vi "Main Tclk.vi"() -> ()   [LabVIEW 2018] (continued)
  in  "Hardware Configuration":T25={"SEM X coil"="SEM-X", "SEM Y coil"="SEM-Y", "FIB X coil"="FIB/ao0", "FIB Y coil"="FIB/ao1", "FIB Detector"="FIB/ai1", "SEM Detectors"="Detectors", "Det min (V)"=-10.0, "Det max (V)"=10.0, "Eanable COM"=TRUE, "COM port"="COM1", "FIB Beam blank"="FIB/port0/line0", "FIB Ext Scan"="FIB/port0/line1", "Det. FIB-NI auto switch"="FIB/port0/line2", "Shutter Drive"="Log/ao0", "Machine Type"=2, "FIB Faraday Cup"="FIB/ai3", "Configuration file"=path "D:/3D FIB-SEM Files/Jeiss.ini", "SEM Max FOV (um)"=350.0, "Machine ID"="Jeiss6/Merlin-xxxx", "Save config file"=FALSE, "Temperature port"="COM3", "Brightness A"=35.0, "Contrast A"=28.0, "Detector B name"="ESB @ 600 V", "Brightness B"=30.0, "Contrast B"=38.0, "Logging Device"="Log"} {"Machine Type" items=["Feiss", "NVision", "Jeiss"]}
  in  "Api":refnum<k7>(container)
  in  "SEM Scan Parameters":T26={"X size (um)"=80.0, "Y size (um)"=80.0, "X center (um)"=0.0, "Y center (um)"=0.0, "X size (V)"=3.2324881417410714, "X size auto"=TRUE, "X stig"=[[0.0]], "Y stig"=[[0.0]], "X aln"=[[0.0]], "Y aln"=[[0.0]], "Scan rate (Hz)"=10000000, "Oversampling"=2, "Oversampling auto"=TRUE, "Frame line rampdown ratio"=0.1, "Pixel size (nm)"=8.0, "WD (mm)"=[[3.0]], "X tiles"=1, "Y tiles"=1, "Overlap (um)"=2.0, "Interlaced"=FALSE, "dX (um)"=[0.0], "dY (um)"=[0.0], "Frames"=1} {"dY (um)" format="%.1f"; "dX (um)" format="%.1f"; "Frames" min=1 step=1; "WD (mm)" step=0.001 format="%.4f"; "Y aln" format="%.1f"; "X aln" format="%.1f"; "Y stig" format="%.1f"; "X stig" format="%.1f"; "Overlap (um)" min=0 step=1; "Y tiles" min=1; "X tiles" min=1; "X size (um)" min=0 format="%.2f"; "Y size (um)" min=0 format="%.2f"; "Frame line rampdown ratio" min=0 max=1 step=0.05 format="%.2g"; "X center (um)" step=1 format="%.3f"; "Y center (um)" step=1 format="%.3f"; "X size (V)" format="%_4g"; "Scan rate (Hz)" max=4000000 step=100000 format="%.2e"; "Pixel size (nm)" min=0.1}
  in  "SEM Options":T27={"GetInfo"=TRUE, "Set Det A para"=TRUE, "Set WD"=FALSE, "Set Mag"=TRUE, "Set stig"=FALSE, "Set aln"=FALSE, "Display"=TRUE, "Save"=TRUE, "8-bit"=FALSE, "Detector A"=TRUE, "Detector B"=TRUE, "Detector C"=FALSE, "Detector D"=FALSE, "Inverse A"=FALSE, "Inverse B"=FALSE, "Inverse C"=FALSE, "Inverse D"=FALSE, "Inverse PNG"=TRUE, "Freeze"=TRUE, "PNG only"=FALSE, "Upload"=FALSE, "Delete after upload"=FALSE}
  in  "Focus Index Options":T28={"Keep aspect ratio"=FALSE, "Show Focus Index"=TRUE, "Focus Index primary grid center"=TRUE, "X Grids"=[[1]], "Y Grids"=[[1]], "Primary X index"=[[1]], "Primary Y index"=[[1]]} {"Y Grids" step=2; "X Grids" step=2}
  out "AS Count":u8 caption="Counts"
  out "AF Count":u8 caption="Counts"
  in  "AS Steps":u8=7
  in  "AS Range (%)":sgl=0.4 min=0 step=1
  in  "Auto Stig":bool
  in  "FI Detector":u16(ring) caption="Detector" items=["A", "B", "C", "D"]
  in  "Auto Focus":bool
  in  "AF Range (nm)":sgl=1800.0 caption="Range" min=0 step=1000
  in  "AF Steps":u8=7 caption="Steps"
  in  "Auto Optimzation":bool=TRUE
  in  "Images per Auto Optimization":u16=200 caption="Auto Optimization Every"
  in  "AA Steps":u8=7
  in  "AA Range (%)":sgl=18.0
  in  "Auto Align":bool
  out "AA Count":u8 caption="Counts"
  in  "Y shift (nm/image)":sgl step=0.1 format="%.1f"
  in  "X shift (nm/image)":sgl step=0.1 format="%.1f"
  in  "Mid Mag SEM":T29={"Mid mag scan"=FALSE, "Prior to main scan"=FALSE, "Mid mag interval"=500, "X size (um)"=200.0, "Y size (um)"=200.0, "X center (um)"=0.0, "Y center (um)"=0.0, "Mid mag scan rate (Hz)"=1000000, "Pixel size (nm)"=10.0, "Show MM box"=TRUE} {"X center (um)" step=1.0 format="%.4f"; "Y center (um)" step=1.0 format="%.4f"; "Mid mag interval" min=1 step=1; "Mid mag scan rate (Hz)" max=4000000 step=100000 format="%.2e"}
  in  "Low Mag SEM":T30={"Low mag scan"=TRUE, "Prior to main scan"=FALSE, "Low mag interval"=1, "Low mag scan FOV (micron)"=300.0, "Low mag scan rate (Hz)"=1000000, "Show HM box"=TRUE} {"Low mag interval" min=1 step=1; "Low mag scan rate (Hz)" max=4000000 step=100000 format="%.2e"; "Low mag scan FOV (micron)" step=50.0}
  out "Mid Mag SEM on":bool
  in  "Manual Upload":bool
  in  "Smart upload":bool=TRUE
  in  "Smart upload FI threshold":u8=75 caption="Threshold"
  in  "Start Current DataLog":bool
  in  "Interval (s)":u16=60
  in  "Start FIB HV DataLog":bool=TRUE
  out "Logging Channels":tag[](array[tag])=["Log/ai0", "Log/ai1", "Log/ai2", "Log/ai3", "Log/ai4", "Log/ai5", "Log/ai6", "Log/ai7", "Log/ai8", "Log/ai9", "Log/ai10", "Log/ai11", "Log/ai12", "Log/ai13", "Log/ai14", "Log/ai15", "Log/ai16", "Log/ai17", "Log/ai18", "Log/ai19", "Log/ai20", "Log/ai21", "Log/ai22", "Log/ai23", "Log/ai24", "Log/ai25", "Log/ai26", "Log/ai27", "Log/ai28", "Log/ai29", "Log/ai30", "Log/ai31"]
  in  "Parameter Names":string[](array[string])=["Faraday Cup Current", "Specimen Current", "Beam Dump 1 Current", "Beam Dump 2 Current"]
  in  "Samples size":u16=100
  out "Log Device":tag="Log"
  in  "Sample rate (Hz)":dbl=1000.0 format="%0.2f"
  in  "Enable logging":bool=TRUE
  out "Active logging channels":string="Log/ai0:3"
  out "Re-read HVDataLog":bool caption="Success"
  out "Logging status before profiling":bool
  in  "File Information":T31={"File path"=path "E:/Images", "Notes"="", "Save recipe"=FALSE, "Load recipe"=FALSE, "Sample ID"=""}
  in  "After SEM":bool=TRUE
  in  "Save Probe Table":bool
  in  "Max FIB probe":bool
  in  "Min FIB probe":bool
  in  "SEM Shutter":bool
  in  "Extractor (kV)":sgl=-6.3 step=0.01 format="%.3f"
  in  "Sweep enabled":bool
  in  "Focus (V)":dbl min=-10.0 max=10.0 step=0.1 format="%.3g"
  in  "Sweep rate (Hz)":dbl=0.5 min=0.01 step=0.1 format="%0.2f"
  in  "Imbalance (V)":dbl min=-10.0 max=10.0 step=0.1 format="%.3g"
  in  "Sweep direction":bool
  in  "Angle (V)":dbl min=-10.0 max=10.0 step=0.1 format="%.3g"
  in  "Position (V)":dbl min=-10.0 max=10.0 step=0.1 format="%.3g"
  in  "Level #":u8
  in  "Sweep #":u8=1 min=1
  in  "FIB Scan Parameters":T32={"X resolution"=512, "Z resolution"=512, "X center"=0.0, "Z center"=0.0, "X size (V)"=16.0, "Z size (V)"=16.0, "Frame line rampdown ratio"=-0.1, "Scan rate (Hz)"=2000000, "Oversampling"=2} {"Z size (V)" min=0.0 max=20.0; "X size (V)" min=0.0 max=20.0; "Frame line rampdown ratio" min=-1.0 max=1.0 step=0.05 format="%.2g"; "Scan rate (Hz)" max=4000000 format="%#.6p"; "Z resolution" max=2048; "X resolution" max=2048}
  in  "FIB Options":T33={"Scan mode"=0, "Flip x"=FALSE, "Flip z"=TRUE, "Det"=0} {"Scan mode" items=["Raster", "Serpentine"]; "Det" items=["Detector A", "Detector B"]}
  in  "Update":bool
  in  "FIB-SEM Angle":dbl=90.0 min=0.0 max=90.0
  in  "FIB Zoom Parameters":T34={"X resolution"=500, "Y resolution"=50, "X center"=0.0, "Y center"=0.0, "X size (V)"=0.0, "Y size (V)"=0.0, "Frame line rampdown ratio"=-0.1, "Scan rate (Hz)"=2000000, "Oversampling"=2} {"Frame line rampdown ratio" min=-1.0 max=1.0 step=0.05 format="%.2g"; "Scan rate (Hz)" max=4000000 format="%#.6p"}
  in  "FIB Bit Size (nm)":dbl
  in  "FIB time lapse (s)":u32=60
  out "FIB file name":path
  in  "SEM-FIB Delay (s)":u32
  in  "FIB Y zoom pixel (nm)":dbl=20.0 caption="Y pixel (nm)" format="%.1f"
  in  "Pre image":bool
  in  "Post image":bool
  out "13nA Condenser (V)":i32=565
  out "27nA Condenser (V)":i32=585
  out "FIB probe switching":string="Go to                 or               current of the same probe "
  out "Fail #":u8
  out "SEM shutter status":string="Unknown"
  in  "FIB Imaging Probe":string(combo)="30kV:50pA ref"
  in  "Damping":bool
  in  "Shtr Tune":bool
  in  "Stop Reheat":bool
  in  "Reheat Parameters":T1={"Filament I (A)"=3.0, "Reheat time (s)"=45.0, "Emission (uA)"=1.5, "Calculate V/I slope"=TRUE, "Pre-calc delay (min)"=5.0, "Disable Reheat Retries"=FALSE, "Restore Voltages"=TRUE} {"Pre-calc delay (min)" format="%.2f"; "Emission (uA)" format="%.1f"; "Filament I (A)" format="%.2f"; "Reheat time (s)" format="%.1f"}
  out "Auto reheat running":bool
  out "Last auto reheat":timestamp
  out "Reheat complete file":path=path "C:/Program Files (x86)/FEI Company/BDS/Reheat/Complete.txt"
  out "Reheat stopped file":path=path "C:/Program Files (x86)/FEI Company/BDS/Reheat/Stopped.txt"
  out "FIB Reheat Log Files":path=path "D:/3D FIB-SEM Files/FIB Reheat Log"
  out "Reheat time":timestamp
  out "Reheat start file":path=path "C:/Program Files (x86)/FEI Company/BDS/Reheat/Start.txt"
  out "Shutter Drive Local?":tag="Log/ao0"
  out "Send reheat start email":bool
  in  "Open FIB gun valve":bool=TRUE caption="Gun Valve"
  out "FIB Gun Valve Status":string="FIB Gun Valve is Open"
  out "FIB Gun State":string="Regulating"
  in  "Request to stop reheat":bool
  in  "Request to reheat":bool
  out "Reheat completed":bool
  in  "Turn FIB gun standby":bool
  in  "Turn off FIB gun":bool
  in  "Turn on FIB gun":bool=TRUE
  out "FIB V/I slope":sgl format="%.1f"
  in  "Get V/I slope":bool
  in  "FIB probe auto min":bool
  in  "FIB Milling Objective (V)":sgl=14275.0
  in  "FIB Profile":bool
  in  "Reset Focus":bool=TRUE
  in  "Mill Stop":bool
  in  "Mill Manual Pause":bool
  in  "Beam blanked":bool
  in  "Spot":bool
  in  "Milling para":T35={"X resolution"=4096, "Z resolution"=125001, "X offset (um)"=0.0, "Z offset (um)"=0.0, "X center (um)"=0.0, "Z center (um)"=0.0, "X size (um)"=250.0, "Z size (um)"=250.0, "UL-Ang"=90.0, "UR-Ang"=90.0, "Line milling time (s)"=5.0, "Z-step (nm)"=8.0, "Lines auto pause"=1, "Auto pause"=FALSE, "Mill from Bottom"=FALSE, "FIB FOV (um)"=500.0, "Auto Profile"=FALSE, "Mill start from Last"=FALSE, "FIB PID on"=FALSE, "FIB PID reset"=FALSE, "FIB PID measured"=0, "FIB PID target"=0.0, "FIB PID target slope"=0.0, "FIB PID P"=0.001, "FIB PID I"=0.01, "FIB PID D"=0.0, "Emission (uA)"=1.36, "Suppressor (V)"=50.0, "Auto reheat"=FALSE} caption="Milling Parameters" {"Suppressor (V)" step=0.1; "Emission (uA)" step=0.1 format="%.2g"; "FIB PID measured" items=["Spec.", "B.D. 1", "B.D. 2", "Mill", "Spec. +"]; "FIB PID target slope" min=-1 max=1 step=0.1; "FIB PID target" step=0.1 format="%.1f"; "UR-Ang" format="%.2f"; "UL-Ang" format="%.2f"; "Z offset (um)" step=0.02 format="%.3g"; "X offset (um)" step=1 format="%.3g"; "FIB FOV (um)" format="%.3g"; "Line milling time (s)" step=0.1 format="%.1f"; "Z center (um)" format="%#.3g"; "X center (um)" format="%#.3g"}
  in  "Mill":bool
  in  "ROI":bool
  in  "Stig Options":enum16{"Defaut", "Stig X", "Stig Y"}(ring)
  in  "Transition time (min)":u16
  in  "PID Target (%)":sgl=100.0 format="%.1f"
  in  "FIB Milling Probe":string(combo)="30kV:50pA ref"
  in  "FIB blank condenser %":u8=50 caption="FIB Condenser @ SEM:" max=100
  in  "Additional Info":cluster{"Restart flag":u8, "Stage move flag":u8}
  in  "Coarse milling":bool
  out "Temperature warning armed":bool
  in  "E-mail test":bool
  out "3D image paused armed":bool=TRUE
  in  "Mail server":string="mail.hhmi.org"
  in  "Email Alert Recipients":string[](array[string])=["xuc@janelia.hhmi.org"]
  out "FIB emission limit warning armed":bool=TRUE
  out "EHT off":bool
  out "SW error warning armed":bool=TRUE
  out "Focus index warning armed":bool=TRUE
  out "Focus index recovery active":bool
  out "Temperature recovery active":bool
  in  "Alert Settings":T36={"3D imaging paused alarm"=TRUE, "FIB emission warning"=TRUE, "Low limit"=1.38, "High limit"=2.0, "Specimen @ SEM alarm"=TRUE, "FIB CL current alarm"=TRUE, "Beam Dump 1 alarm"=TRUE, "Milling Z voltage alarm"=TRUE, "EHT off alarm"=TRUE, "Detector over scale warning"=TRUE, "Image clipping alarm"=FALSE, "Warning limit (um)"=1.5, "Stop limit (um)"=0.5, "Temperature alarm"=TRUE, "Pause 3D-ING"=FALSE, "Low limit (F)"=65.0, "High limit (F)"=80.0, "Temp limit auto"=TRUE, "Delta (F)"=0.2, "Gradient limit (F/min)"=0.03, "SW error warning"=TRUE, "Focus index warning"=TRUE, "Focus index low limit"=0.1, "Focus index stop limit"=0.0, "Run Auto Stig"=FALSE, "FI low limit auto"=TRUE, "FI stop limit auto"=TRUE} {"Stop limit (um)" format="%.2f"; "Warning limit (um)" format="%.2f"; "Focus index stop limit" format="%_3g"; "Focus index low limit" format="%_3g"; "High limit (F)" format="%.2g"; "Low limit (F)" format="%.2g"; "High limit" format="%.2f"; "Low limit" format="%.2f"}
  out "Reheat warning armed":bool=TRUE
  out "Email Log Files":path=path "D:/3D FIB-SEM Files/Email Log"
  out "Initial Options":T27={"GetInfo"=TRUE, "Set Det A para"=TRUE, "Set WD"=FALSE, "Set Mag"=TRUE, "Set stig"=FALSE, "Set aln"=FALSE, "Display"=TRUE, "Save"=TRUE, "8-bit"=TRUE, "Detector A"=TRUE, "Detector B"=TRUE, "Detector C"=FALSE, "Detector D"=FALSE, "Inverse A"=FALSE, "Inverse B"=FALSE, "Inverse C"=FALSE, "Inverse D"=FALSE, "Inverse PNG"=TRUE, "Freeze"=TRUE, "PNG only"=TRUE, "Upload"=TRUE, "Delete after upload"=FALSE}
  in  "Scan xn":bool
  out "Status message":string="API Initialized"
  in  "FIB":bool
  out "COM port":refnum<visa-resource-name>="COM1"
  in  "Image Tabs":T37(tab)=enum."Auto Focus / Stig / Align"
  out "Det B LM":i16[][](graph)
  out "Det A LM":i16[][](graph)
  out "Det B":i16[][](graph)
  out "Det A":i16[][](graph)
  out "Low res scale tiled":dbl[][](array[numeric])
  in  "Tiled Image fit to":u8(ring) items=["Width", "Height"]
  out "Det A over scale":bool caption="Over scale"
  out "Det B over scale":bool caption="Over scale"
  out "DetA e- Scaling":sgl caption="Electon # Scaling" format="%.3g"
  out "Detector A":i16[][](graph) caption="InLens"
  out "Detector B":i16[][](graph) caption="ESB @ 600 V"
  out "DetB e- Scaling":sgl caption="Electon # Scaling" format="%.3g"
  out "Detector A Low Mag":i16[][](graph)
  out "Detector B Low Mag":i16[][](graph)
  out "FIB Image":i16[][](graph)
  out "Faraday Cup RT":sgl caption="Faraday Cup" format="%.3g"
  out "Specimen RT":sgl=5.58914 caption="Specimen" format="%.3g"
  out "BD1 RT":sgl=5.6069436 caption="Beam Dump" format="%.3g"
  out "BD2 RT":sgl=5.6180186 format="%.3g"
  out "Cursor Z (V)":dbl format="%.4g"
  out "Post Image":i16[][](graph)
  out "Pre Image":i16[][](graph)
  out "FIB Y zoom size (um)":dbl caption="Y size (um)" format="%.3g"
  out "FIB X zoom size (um)":dbl caption="Y size (um)" format="%.3g"
  out "AAX Success tiled":bool[][](array[boolean]) caption="Success"
  out "AAY Y tile":u8 caption="Y" min=1
  out "AAY X tile":u8 caption="X" min=1
  out "ASY Y tile":u8 caption="Y" min=1
  out "ASY X tile":u8 caption="X" min=1
  out "AAX Y tile":u8 caption="Y" min=1
  out "AAX X tile":u8 caption="X" min=1
  out "ASX Y tile":u8 caption="Y" min=1
  out "ASX X tile":u8 caption="X" min=1
  out "AF Y tile":u8 caption="Y" min=1
  out "AF X tile":u8 caption="X" min=1
  out "Auto Aln Y":T38(graph)
  out "Auto Aln X":T38(graph)
  out "Dynamic Focus":cluster{cluster{sgl, "Numeric":dbl}[]}[](graph)
  out "Auto Stig Y":T38(graph)
  out "Auto Stig X":T38(graph)
  out "FI array":sgl[](array[numeric])
  out "Auto Focus Graph":T38(graph)
  out "FI grid array":sgl[][][](array[numeric])
  out "WD array tiled":sgl[][][](array[numeric])
  out "AF Success tiled":bool[][](array[boolean]) caption="Success"
  out "ASX Success tiled":bool[][](array[boolean]) caption="Success"
  out "ASY Success tiled":bool[][](array[boolean]) caption="Success"
  out "AAY Success tiled":bool[][](array[boolean]) caption="Success"
  out "Best WD (mm) tiled":dbl[][](array[numeric]) caption="Best WD (mm)" format="%.4g"
  out "Best WD FI tiled":dbl[][](array[numeric]) format="%#_3g"
  out "Best Stig X (%) tiled":dbl[][](array[numeric]) caption="Best Stig X (%)" format="%.2g"
  out "Best Stig X FI tiled":dbl[][](array[numeric]) format="%#_3g"
  out "Best Stig Y (%) tiled":dbl[][](array[numeric]) caption="Best Stig Y (%)" format="%.2g"
  out "Best Stig Y FI tiled":dbl[][](array[numeric]) format="%#_3g"
  out "Best Aln X (%) tiled":dbl[][](array[numeric]) caption="Best Aln X (%)" format="%.2g"
  out "Best Aln X FI tiled":dbl[][](array[numeric]) format="%#_3g"
  out "Best Aln Y (%) tiled":dbl[][](array[numeric]) caption="Best Aln Y (%)" format="%.2g"
  out "Best Aln Y FI tiled":dbl[][](array[numeric]) format="%#_3g"
  out "Slope tiled":dbl[][](array[numeric]) caption="Slope" format="%#_4g"
  out "Focus index log":cluster{u32[], "Focus index array":sgl[]}[](graph)
  out "Delta X log":T39(graph)
  out "Delta Z log":T40(graph)
  out "Delta Y log":T41(graph)
  out "Beam Dump log":cluster{u32[], "BD1 low limit array":sgl[]}[](graph)
  out "Specimen I log":cluster{u32[], "SEM Specimen I array":sgl[]}[](graph)
  out "Faraday Cup log":cluster{u32[], "Temp low limit array":sgl[]}[](graph)
  out "Temp log":cluster{u32[], "Temp array":sgl[]}[](graph)
  out "Log time array":u32[](array[numeric])
  out "FIB HV DataLog":cluster{sgl, sgl}(graph)={849.284, 1.5152843}
  out "Measurements":sgl[][](graph)=[[0.0, 0.0, 0.0, 0.0, 0.0, 0.0, 0.0, 0.0, 0.0, 0.0, 0.0, 0.0, 0.0, 0.0, 0.0, 0.0, 0.0, 0.0, 0.0, 0.0, 0.0, 0.0, 0.0, 0.0, 0.0, 0.0, 0.0, 0.0, 0.0, 0.0, 0.0, 0.0, 0.0, 0.0, 0.0, 0.0, 0.0, 0.0, 0.0, 0.0, 0.0, 0.0, 0.0, 0.0, 0.0, 0.0, 0.0, 0.0, 0.0, 0.0, 0.0, 0.0, 0.0, 0.0, 0.0, 0.0, 0.0, 0.0, 0.0, 0.0, 0.0, 0.0, 0.0, 0.0, 0.0, 0.0, 0.0, 0.0, 0.0, 0.0, 0.0, 0.0, 0.0, 0.0, 0.0, 0.0, 0.0, 0.0, 0.0, 0.0, 0.0, 0.0, 0.0, 0.0, 0.0, 0.0, 0.0, 0.0, 0.0, 0.0, 0.0, 0.0, 0.0, 0.0, 0.0, 0.0, 0.0, 0.0, 0.0, 0.0], [5.6226387, 5.0222063, 5.522835, 5.619419, 5.61137, 5.606541, 5.603322, 5.603322, 5.603322, 5.600102, 5.603322, 5.604931, 5.6017118, 5.600102, 5.600102, 5.596883, 5.6017118, 5.5984926, 5.5984926, 5.5984926, 5.5984926, 5.600102, 5.5984926, 5.5984926, 5.600102, 5.5984926, 5.5984926, 5.600102, 5.595273, 5.596883, 5.5984926, 5.595273, 5.600102, 5.595273, 5.595273, 5.595273, 5.595273, 5.593663, 5.593663, 5.595273, 5.593663, 5.5920534, 5.595273, 5.5920534, 5.595273, 5.596883, 5.595273, 5.595273, 5.595273, 5.593663, 5.595273, 5.596883, 5.595273, 5.593663, 5.593663, 5.593663, 5.596883, 5.593663, 5.5920534, 5.593663, 5.5920534, 5.593663, 5.5920534, 5.5920534, 5.593663, 5.5904436, 5.5920534, 5.593663, 5.5904436, 5.593663, 5.595273, 5.5920534, 5.5920534, 5.593663, 5.5904436, 5.5920534, 5.5904436, 5.5920534, 5.5904436, 5.5904436, 5.5920534, 5.5920534, 5.5920534, 5.5904436, 5.5920534, 5.5920534, 5.5872245, 5.595273, 5.5904436, 5.5904436, 5.5904436, 5.5920534, 5.588834, 5.5904436, 5.5904436, 5.5920534, 5.5920534, 5.5904436, 5.588834, 5.5904436], [6.6013584, 5.604931, 5.519615, 5.5920534, 5.608151, 5.608151, 5.606541, 5.608151, 5.604931, 5.604931, 5.606541, 5.603322, 5.6017118, 5.603322, 5.6017118, 5.603322, 5.604931, 5.603322, 5.603322, 5.603322, 5.6017118, 5.6017118, 5.603322, 5.600102, 5.600102, 5.603322, 5.5984926, 5.596883, 5.6017118, 5.596883, 5.5984926, 5.600102, 5.600102, 5.6017118, 5.600102, 5.5984926, 5.6017118, 5.5984926, 5.596883, 5.5984926, 5.596883, 5.5984926, 5.596883, 5.600102, 5.596883, 5.595273, 5.595273, 5.5984926, 5.596883, 5.596883, 5.595273, 5.5984926, 5.5984926, 5.5984926, 5.5984926, 5.595273, 5.596883, 5.593663, 5.596883, 5.593663, 5.595273, 5.5984926, 5.595273, 5.595273, 5.593663, 5.593663, 5.596883, 5.595273, 5.593663, 5.595273, 5.596883, 5.593663, 5.593663, 5.5920534, 5.595273, 5.596883, 5.596883, 5.595273, 5.593663, 5.5920534, 5.593663, 5.593663, 5.5904436, 5.595273, 5.593663, 5.593663, 5.5920534, 5.593663, 5.593663, 5.5920534, 5.5920534, 5.593663, 5.5920534, 5.5920534, 5.593663, 5.593663, 5.5920534, 5.595273, 5.593663, 5.595273], [6.177998, 5.91883, 5.6274676, 5.6097603, 5.6178093, 5.619419, 5.6178093, 5.6178093, 5.61459, 5.6161995, 5.61459, 5.61298, 5.6178093, 5.6161995, 5.61459, 5.6161995, 5.61459, 5.6161995, 5.61298, 5.61298, 5.61137, 5.61137, 5.61459, 5.61137, 5.61137, 5.61137, 5.61298, 5.6097603, 5.61298, 5.61298, 5.61459, 5.61298, 5.61137, 5.608151, 5.61459, 5.608151, 5.6097603, 5.6097603, 5.608151, 5.61137, 5.61137, 5.608151, 5.61298, 5.608151, 5.608151, 5.608151, 5.6097603, 5.608151, 5.606541, 5.604931, 5.6097603, 5.61137, 5.6097603, 5.604931, 5.608151, 5.6097603, 5.606541, 5.6097603, 5.608151, 5.606541, 5.604931, 5.6097603, 5.604931, 5.608151, 5.6097603, 5.608151, 5.606541, 5.604931, 5.608151, 5.606541, 5.606541, 5.604931, 5.606541, 5.606541, 5.6097603, 5.604931, 5.606541, 5.604931, 5.604931, 5.603322, 5.604931, 5.603322, 5.606541, 5.603322, 5.603322, 5.603322, 5.603322, 5.603322, 5.604931, 5.606541, 5.604931, 5.603322, 5.603322, 5.606541, 5.604931, 5.603322, 5.603322, 5.606541, 5.6017118, 5.603322]]
  in  "Clear":bool
  in  "Stop":bool
  in  "Scan x1":bool
  # "Direction"
  # "Start\nfrom"
  # "<"
  # "Grids"
  # "Primary"
  # "Recipe"
  # "Det"
  # "after"
  # "Detector A"
  # "Images"
  # "nm"
  # "%"
  # "%"
  # "Direction"
  # "Start\nfrom"
  # "<"
  # "Grids"
  # "Primary"
  # "Det"
  # "after"
  # "Recipe"
  # "Brightness & Contrast (%)"
  # "Detector A"
  # "Brightness & Contrast (%)"
  # "Brightness & Contrast (%)"
  # "Detector A"
  # "Brightness & Contrast (%)"
  # "Currents (nA)"
  # "/"
  # "line(s)"
  # "% of"
  # "%"
  # "Hz"
  # "Scanning time"
  # "m"
  # "s"
  # "Remaining time"
  # "m"
  # "s"
  # "Cycle time (s)"
  # "@"
  # "Scan coils"
  # "Detector"
  # "Brightness & Contrast (%)"
  # "A       InLens"
  # "Images"
  # "nm"
  # "%"
  # "%"
  # "Det"
  # "after"
  # "Grids"
  # "Primary"
  # "% of FI alarm limit"
  # "Recipe"
  # "FIB Zoom Image"
  # "Flip"
  # "recovers in"
  # "min"
  # "% during Milling"
  # "Direction"
  # "Start\nfrom"
  # "@"
  # "<"
  # "or"
  # "<"
  # "Det"
  # "Images fit to"
  # "Images fit to"
  # "Images fit to"
  # "X"
  # "um"
  # ":"
  # "%"
  # ":"
  # ":"
  # ":"
  # ":"
  # "Faraday Cup"
  # "Specimen"
  # "Beam Dump"
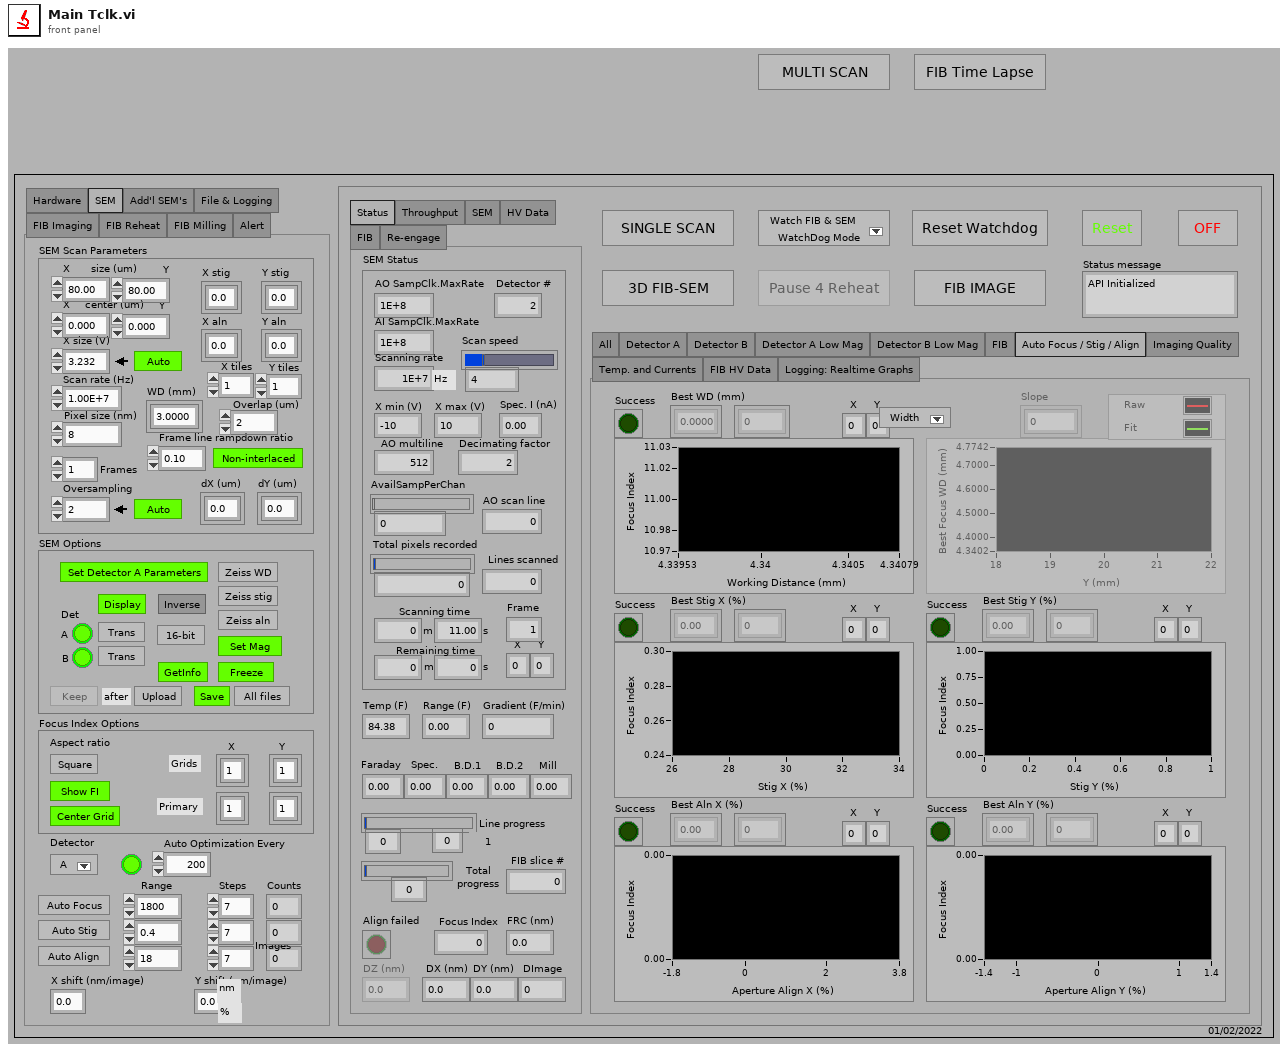
[diagram p1: front panel]
types:
  T1 = cluster{"Filament I (A)":sgl, "Reheat time (s)":sgl, "Emission (uA)":sgl, "Calculate V/I slope":bool, "Pre-calc delay (min)":sgl, "Disable Reheat Retries":bool, "Restore Voltages":bool}
  T2 = cluster{"3D imaging paused alarm":bool, "FIB emission limit warning":bool, "Low limit":dbl, "High limit":dbl, "Specimen @ SEM alarm":bool, "Specimen @ FIB alarm ":bool, "Beam Dump 1 alarm":bool, "Milling Z voltage alarm":bool, "EHT off alarm":bool, "Detector over scale warning":bool, "Image clipping alarm":bool, "Warning limit (um)":sgl, "Stop limit (um)":sgl, "Temperature alarm":bool, "Pause 3D-ING":bool, "Low limit (F)":sgl, "High limit (F)":sgl, "Temp limit auto":bool, "Delta (F)":sgl, "Gradient limit (F/min)":sgl, "SW error warning":bool, "Focus index warning":bool, "Focus index low limit":sgl, "Focus index stop limit":sgl, "Run Auto Stig":bool, "FI low limit auto":bool, "FI stop limit auto":bool}
  T3 = cluster{"dWD":sgl[][], "dX stig":sgl[][], "dY stig":sgl[][], "dX aln":sgl[][], "dY aln":sgl[][], "dX (um)":sgl[], "dY (um)":sgl[]}
  T4 = cluster{cluster{"Center":dbl, "A Img Focus Index":dbl}[]}[][][]
  T5 = cluster{"X size (um)":sgl, "Y size (um)":sgl, "X center (um)":dbl, "Y center (um)":dbl, "X size (V)":dbl, "X size auto":bool, "X stig":sgl[][], "Y stig":sgl[][], "X aln":sgl[][], "Y aln":sgl[][], "Scan rate (Hz)":u32, "Oversampling":u32, "Oversampling auto":bool, "Frame line rampdown ratio":sgl, "Pixel size (nm)":sgl, "WD (mm)":sgl[][], "X tiles":u8, "Y tiles":u8, "Overlap (um)":sgl, "Interlaced":bool, "dX (um)":sgl[], "dY (um)":sgl[], "Frames":u8}
  T6 = cluster{"HW Config":cluster{"SEM X coil":refnum<k15>, "SEM Y coil":refnum<k15>, "Detectors":refnum<k15>, "Det min (V)":dbl, "Det max (V)":dbl, "Eanable COM":bool, "COM port":refnum<visa-resource-name>, "Detector FIB-NI auto switch":tag, "Machine Type":u8, "Machine ID":string, "SEM Max FOV (um)":sgl}, "Det Info":cluster{"Brightness A":dbl, "Contrast A":dbl, "Detector B name":string, "Brightness B":dbl, "Contrast B":dbl, "Detector C name":string, "Detector D name":string}, "SEM Scan Parameters":cluster{"X size (um)":sgl, "Y size (um)":sgl, "X center (um)":dbl, "Y center (um)":dbl, "X size (V)":dbl, "X size auto":bool, "X stig":sgl[][], "Y stig":sgl[][], "X aln":sgl[][], "Y aln":sgl[][], "Scan rate (Hz)":u32, "Oversampling":u32, "Oversampling auto":bool, "Frame line rampdown ratio":sgl, "Pixel size (nm)":sgl, "WD (mm)":sgl[][], "X tiles":u8, "Y tiles":u8, "Overlap (um)":sgl, "Interlaced":bool, "dX (um)":sgl[], "dY (um)":sgl[], "Frames":u8}, "SEM Options":cluster{"GetInfo":bool, "Set Det A para":bool, "Set WD":bool, "Set Mag":bool, "Set stig":bool, "Set aln":bool, "Display":bool, "Save":bool, "8-bit":bool, "Detector A":bool, "Detector B":bool, "Detector C":bool, "Detector D":bool, "Inverse A":bool, "Inverse B":bool, "Inverse C":bool, "Inverse D":bool, "Inverse PNG":bool, "Freeze":bool, "PNG only":bool, "Upload":bool, "Delete after upload":bool}, "Focus Index Options":cluster{"Keep aspect ratio":bool, "Show Focus Index":bool, "Focus Index primary grid center":bool, "X Grids":u8[][], "Y Grids":u8[][], "Primary X index":u8[][], "Primary Y index":u8[][]}, "File Information":cluster{"File path":path, "Notes":string, "Save recipe":bool, "Load recipe":bool, "Sample ID":string}, "Milling para":cluster{"X resolution":u32, "Y resolution":u32, "X offset (um)":sgl, "Y offset (um)":sgl, "X center (um)":sgl, "Y center (um)":sgl, "X size (um)":sgl, "Y size (um)":sgl, "UL-Ang":sgl, "UR-Ang":sgl, "Line milling time (s)":sgl, "Z-step (nm)":dbl, "Lines auto pause":u16, "Auto pause":bool, "Mill from Bottom":bool, "FIB FOV (um)":sgl, "Auto Profile":bool, "Mill start from Last":bool, "FIB PID on":bool, "FIB PID reset":bool, "FIB PID measured":u8, "FIB PID target":sgl, "FIB PID target slope":sgl, "FIB PID P":sgl, "FIB PID I":sgl, "FIB PID D":sgl, "Emission (uA)":dbl, "Suppressor (V)":sgl, "Auto reheat":bool}, "Additional Info":cluster{"Restart flag":u8, "Stage move flag":u8}}
  T7 = cluster{"SEM Scan Parameters":cluster{"X size (um)":sgl, "Y size (um)":sgl, "X center (um)":dbl, "Y center (um)":dbl, "X size (V)":dbl, "X size auto":bool, "X stig":sgl[][], "Y stig":sgl[][], "X aln":sgl[][], "Y aln":sgl[][], "Scan rate (Hz)":u32, "Oversampling":u32, "Oversampling auto":bool, "Frame line rampdown ratio":sgl, "Pixel size (nm)":sgl, "WD (mm)":sgl[][], "X tiles":u8, "Y tiles":u8, "Overlap (um)":sgl, "Interlaced":bool, "dX (um)":sgl[], "dY (um)":sgl[], "Frames":u8}, "Detector Information":cluster{"Brightness A":dbl, "Contrast A":dbl, "Detector B name":string, "Brightness B":dbl, "Contrast B":dbl, "Detector C name":string, "Detector D name":string}, "SEM Options":cluster{"GetInfo":bool, "Set Det A para":bool, "Set WD":bool, "Set Mag":bool, "Set stig":bool, "Set aln":bool, "Display":bool, "Save":bool, "8-bit":bool, "Detector A":bool, "Detector B":bool, "Detector C":bool, "Detector D":bool, "Inverse A":bool, "Inverse B":bool, "Inverse C":bool, "Inverse D":bool, "Inverse PNG":bool, "Freeze":bool, "PNG only":bool, "Upload":bool, "Delete after upload":bool}, "Focus Index Options":cluster{"Keep aspect ratio":bool, "Show Focus Index":bool, "Focus Index primary grid center":bool, "X Grids":u8[][], "Y Grids":u8[][], "Primary X index":u8[][], "Primary Y index":u8[][]}, "Image fit to":u8, "File Information":cluster{"File path":path, "Notes":string, "Save recipe":bool, "Load recipe":bool, "Sample ID":string}, "Low mag SEM":cluster{"Low mag scan":bool, "Prior to main scan":bool, "Low mag interval":u32, "Low mag scan FOV (micron)":dbl, "Low mag scan rate (Hz)":u32, "Show HM box":bool}, "Mid Mag SEM":cluster{"Mid mag scan":bool, "Prior to main scan":bool, "Mid mag interval":u32, "X size (um)":sgl, "Y size (um)":sgl, "X center (um)":dbl, "Y center (um)":dbl, "Mid mag scan rate (Hz)":u32, "Pixel size (nm)":dbl, "Show MM box":bool}, "FIB-SEM Angle":dbl, "Milling para":cluster{"X resolution":u32, "Z resolution":u32, "X offset (um)":sgl, "Z offset (um)":sgl, "X center (um)":sgl, "Z center (um)":sgl, "X size (um)":sgl, "Z size (um)":sgl, "UL-Ang":sgl, "UR-Ang":sgl, "Line milling time (s)":sgl, "Z-step (nm)":dbl, "Lines auto pause":u16, "Auto pause":bool, "Mill from Bottom":bool, "FIB FOV (um)":sgl, "Auto Profile":bool, "Mill start from Last":bool, "FIB PID on":bool, "FIB PID reset":bool, "FIB PID measured":u8, "FIB PID target":sgl, "FIB PID target slope":sgl, "FIB PID P":sgl, "FIB PID I":sgl, "FIB PID D":sgl, "Emission (uA)":dbl, "Suppressor (V)":sgl, "Auto reheat":bool}, "FI Detector":u16, "Auto Optimzation":bool, "Images per Auto Optimization":u16, "AF Range (nm)":dbl, "AF Steps":u8, "AS Range (%)":dbl, "AS Steps":u8, "AA Range (%)":sgl, "AA Steps":u8, "X shift (nm/frame)":dbl, "Y shift (nm/frame)":dbl, "FIB Y zoom pixel (nm)":dbl, "Mail server":string, "Email Alert Recipents":string[], "Alert Settings":cluster{"3D imaging paused alarm":bool, "FIB emission limit warning":bool, "Low limit":sgl, "High limit":sgl, "Specimen @ SEM alarm":bool, "FIB CL current alarm":bool, "Beam Dump 1 alarm":bool, "Milling Z voltage alarm":bool, "EHT off alarm":bool, "Detector over scale warning":bool, "Image clipping alarm":bool, "Warning limit (um)":sgl, "Stop limit (um)":sgl, "Temperature alarm":bool, "Pause 3D-ING":bool, "Low limit (F)":sgl, "High limit (F)":sgl, "Temp limit auto":bool, "Delta (F)":sgl, "Gradient limit (F/min)":sgl, "SW error warning":bool, "Focus index warning":bool, "Focus index low limit":sgl, "Focus index stop limit":sgl, "Run Auto Stig":bool, "FI low limit auto":bool, "FI stop limit auto":bool}, "Reheat Parameters":cluster{"Filament I (A)":sgl, "Reheat time (s)":sgl, "Emission (uA)":sgl, "Calculate V/I slope":bool, "Pre-calc delay (min)":sgl, "Disable Reheat Retries":bool, "Restore Voltages":bool}, "Start FIB HV DataLog":bool, "Interval (s)":u16}
  T8 = cluster{"Brightness A":dbl, "Contrast A":dbl, "Detector B name":string, "Brightness B":dbl, "Contrast B":dbl, "Detector C name":string, "Detector D name":string}
  T9 = cluster{"SEM X coil":refnum<k15>, "SEM Y coil":refnum<k15>, "Detectors A&B":refnum<k15>, "Det min (V)":dbl, "Det max (V)":dbl, "Eanable COM":bool, "COM port":refnum<visa-resource-name>, "Detector FIB-NI auto switch":tag, "Machine Type":u8, "Machine ID":string, "SEM Max FOV (um)":sgl}
  T10 = enum16{"SEM", "FIB", "Milling", "SEM + FIB", "Mill + SEM", "SEM Drift Correction", "FIB Drift Correction", "No Beam", "External", "External + SEM"}
  T11 = enum32{"Status", "Throughput", "SEM", "HV Data", "FIB", "Re-engage"}
  T12 = cluster{"AO SampClk.MaxRate":dbl, "AI SampClk.MaxRate":dbl, "AO rate":dbl, "Scan speed":u8, "Detector #":u8, "X min (V)":dbl, "X max (V)":dbl, "X min index":i32, "X max index":i32, "AO multiline":u32, "Decimating factor":u16, "AvailSampPerChan":u32, "AO scan line":u32, "Total pixels recorded":i32, "Lines scanned":i32, "Scan time (m)":dbl, "Scan time (s)":dbl, "Remaining time (m)":u16, "Remaining time (s)":u8, "SEM Spec. I (nA)":sgl, "Frame":u8, "X tile":u8, "Y tile":u8}
  T13 = cluster{"Detector A":string, "Detector B":string, "Brightness A":sgl, "Contrast A":sgl, "Brightness B":sgl, "Contrast B":sgl, "Magnification":sgl, "Pixel size":sgl, "Working distance":sgl, "EHT":sgl, "Aperture":u8, "High current mode":u8, "Probe current":sgl, "Scan rotation":sgl, "Chamber vac":sgl, "Gun vac":sgl, "Beam shift X":sgl, "Beam shift Y":sgl, "Stig X":sgl, "Stig Y":sgl, "Alignment X":sgl, "Alignment Y":sgl, "Stage X":sgl, "Stage Y":sgl, "Stage Z":sgl, "Stage T":sgl, "Stage R":sgl, "Stage M":sgl}
  T14 = cluster{"A Img Focus Index":sgl, "B Img Focus Index":sgl, "C Img Focus Index":sgl, "D Img Focus Index":sgl}
  T15 = cluster{"A Img Focus Index array":dbl[][], "B Img Focus Index array":dbl[][], "C Img Focux Index array":dbl[][], "D Img Focus Index array":dbl[][]}
  T16 = cluster{"Ext Target (V)":sgl, "Ext Actual (V)":sgl, "Fil Age (hr)":sgl, "Ext I Actual (uA)":sgl, "Fil I Target (A)":sgl, "Fil I Actual (A)":sgl, "Liner Target (V)":sgl, "Liner Actual (V)":sgl, "EHT Target (V)":sgl, "EHT Actual (V)":sgl, "Supp Actual (V)":sgl, "Supp Monitor (V)":sgl, "Gun Vac (Torr)":sgl, "Sys Vac (Torr)":sgl}
